vi "uPublisher Publish.vi"(8 "error in (no error)":errorcluster, 10 "uMsg":refnum<class "uMsg.lvclass">, 11 "uClient_Publisher in":refnum<class "uClient_Publisher.lvclass">) -> (0 "error out":errorcluster, 3 "uClient_Publisher out":refnum<class "uClient_Publisher.lvclass">)   [LabVIEW 2021, in "uFramework.lvlib" / "uClient_Publisher.lvclass"]
doc: "Publish an event to the broker.\nFor optimal performance in high-throughput streaming applications, make sure to set a valid timestamp when creating the message to be published."
uses:
  uClient_Publisher.lvclass
  uMsg/uMsg.lvclass
  uClient_Publisher.lvclass/uClient_Publisher.ctl
  uMsg/uMsg.lvclass/uMsg.ctl
  Bin/uData.lvlibp/uData.lvclass
  Bin/uStringManipulation.lvlibp/uStringManipulation.lvclass
  uTransport/uTransport.lvclass
  U:/Projects/uFramework/Src/uFramework/uClient/uClient.lvclass
  U:/Projects/uFramework/Src/uFramework/uClient_Publisher/uClient_Publisher.lvclass
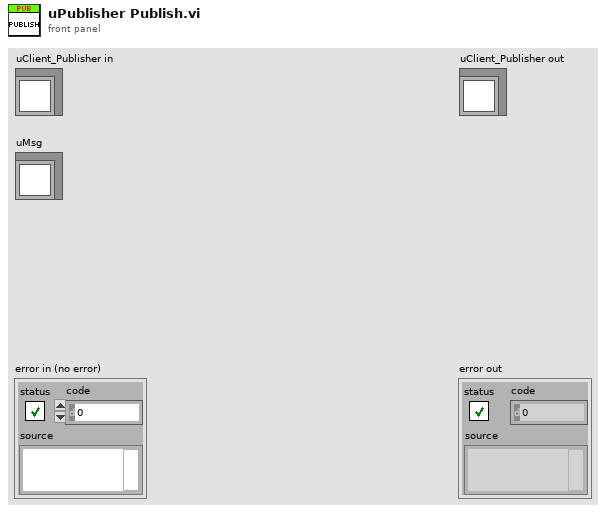
[diagram p1: front panel]
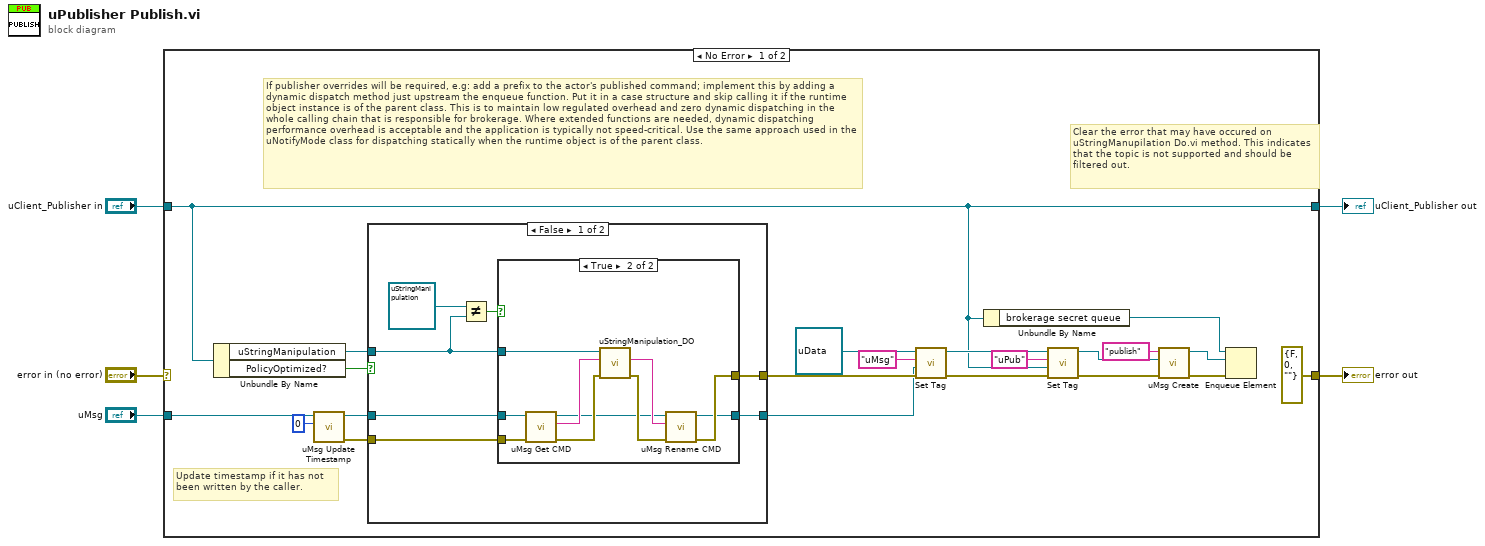
[diagram p0: block diagram]
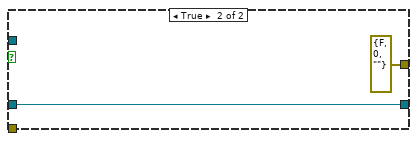
[diagram p3: hidden frame]
diagram:
  n1 = case shown="No Error" "error in (no error)" {
    selector: "error in (no error)" -> [_ w48]
    tunnel: [errorcluster {"status"=FALSE, "code"=0, "source"=""} ("error IO") w48] -> w5
    tunnel: "uClient_Publisher in" -> [w14 w49]
    tunnel: "uMsg" -> [w7 _]
    tunnel: [w14 w49] -> w2
    frame No Error {
      # "Update timestamp if it has not been written by the caller."
      # "Clear the error that may have occured on uStringManupilation Do.vi method. This indicates that the topic is not supported and should be filtered out."
      # "If publisher overrides will be required, e.g: add a prefix to the actor's published command; implement this by adding a dynamic dispatch method just upstream the enqueue function. Put it in a case structure and skip calling it if the runtime object instance is of the parent class. This is to maintain low regulated overhead and zero dynamic dispatching in the whole calling chain that is responsible for brokerage. Where extended functions are needed, dynamic dispatching performance overhead is acceptable and the application is typically not speed-critical. Use the same approach used in the uNotifyMode class for dispatching statically when the runtime object is of the parent class."
      n2 = Unbundle By Name(w14) -> ("uStringManipulation"=w15:refnum<class "uStringManipulation.lvclass">, "PolicyOptimized?"=w10:bool)
      n3 = call "uMsg Update Timestamp.vi"("Timestamp"=u32 0, "uMsg in"=w7) -> ("error out"=w6:errorcluster, "uMsg out"=w8:refnum<class "uMsg.lvclass">)  [unwired: 8 in]
      n4 = case shown="False" w10 {
        tunnel: [w33 errorcluster {"status"=FALSE, "code"=0, "source"=""} ("error out")] -> w17
        tunnel: [w32 w47] -> w16
        tunnel: w15 -> [w29 _]
        tunnel: w8 -> [w28 w47]
        tunnel: w6 -> [w27 _]
        frame False {
          n5 = Not Equal?(x=refnum<class "uStringManipulation.lvclass"> refnum ("uFramework.lvlib:uStringManipulation.lvclass"), y=w29) -> (x != y?=w30:bool)
          n6 = case shown="True" w30 {
            tunnel: w29 -> [_ w45]
            tunnel: [w35 w44] -> w33
            tunnel: w28 -> [w34 w41]
            tunnel: [w34 w42] -> w32
            tunnel: w27 -> [w35 w37]
            frame False {
              # "Avoid the unnecessary dynamic dispatch uStringManipulation method's overhead  if there is no translation provided."
            }
            frame True {
              n7 = call "uMsg Get CMD.vi"("error in (no error)"=w37, "uMsg in"=w41) -> ("error out"=w40:errorcluster, "CMD"=w38:string, "uMsg out"=w36:refnum<class "uMsg.lvclass">)  [unwired: 7 in]
              n8 = call-dynamic "uStringManipulation_DO.vi"("error in (no error)"=w40, "String in"=w38, "uStringManipulation in"=w45) -> ("error out"=w39:errorcluster, "String"=w43:string)  [unwired: 6 in, 1 out]
              n9 = call "uMsg Rename CMD.vi"("error in (no error)"=w39, "New CMD"=w43, "uMsg in"=w36) -> ("error out"=w44:errorcluster, "uMsg out"=w42:refnum<class "uMsg.lvclass">)  [unwired: 7 in]
            }
          }
        }
        frame True {
        }
      }
      n10 = call "Set Tag.vi"("error in (no error)"=w17, "Variant"=w16, "tag (case insensitive)"="uMsg", "uData in"=refnum<class "uData.lvclass"> refnum) -> ("error out"=w23:errorcluster, "uData out"=w21:refnum<class "uData.lvclass">)  [unwired: 5 in, 1 out]
      n11 = Unbundle By Name(w14) -> ("brokerage secret queue"=w25:refnum<queue>)
      n12 = call "Set Tag.vi"("error in (no error)"=w23, "Variant"=w14, "tag (case insensitive)"="uPub", "uData in"=w21) -> ("error out"=w26:errorcluster, "uData out"=w18:refnum<class "uData.lvclass">)  [unwired: 5 in, 1 out]
      n13 = call "uMsg Create.vi"("error in (no error)"=w26, "Payload"=w18, "CMD"="publish") -> ("error out"=w11:errorcluster, "uMsg out"=w12:refnum<class "uMsg.lvclass">)  [unwired: 7 in]
      n14 = Enqueue Element(queue=w25, element=w12, error in (no error)=w11) -> ()  [unwired: 1 in, 3 out]
    }
    frame Error {
    }
  }
  "error out" <- w5
  "uClient_Publisher out" <- w2
